vi "警报.vi"(8 "error in (no error)":errorcluster caption="错误输入（无错误）", 9 "Enable":bool=TRUE caption="启用", 10 "Message":string="警报！请处理仓库环境！" caption="消息") -> (0 "error out":errorcluster caption="错误输出", 2 "确定":bool)   [LabVIEW 2014]
doc: "创建含有警告或用户消息的标准对话框。\n--------------------\n\n该Express VI配置如下:\n\n消息: 警报！请处理仓库环境！"
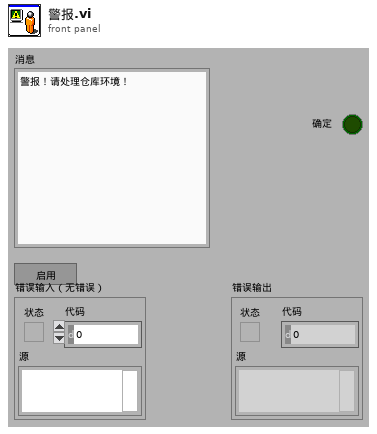
[diagram p1: front panel]
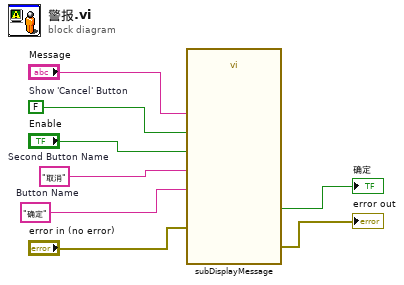
[diagram p0: block diagram]
diagram:
  w3 = "确定"  # Button Name
  w4 = "取消"  # Second Button Name
  w6 = FALSE  # Show 'Cancel' Button
  n1 = call <vilib>:"subDisplayMessage.vi"("Second Button Name"=w4, "Button Name"=w3, "error in (no error)"="error in (no error)", "Enable Message"="Enable", "Show 'Cancel' Button"=w6, "Message to Display"="Message") -> ("error out"=→"error out":errorcluster, "OK?"=→"确定":bool)  [unwired: 4 in]
